vi "myBOT_Draw.vi"(11 "myBOT-Position and Angle":dbl[](array[numeric])) -> (3 "myBOT-Scene":refnum<vi>)   [LabVIEW 2013]
doc: "\"myBOT_Draw.vi\": Draws the myBOT on a 3D Picture Control.\nThis VI has two functions:\n1) The first time the VI is called, CAD Data are gathered, different objects are identified and placed on the 3D Picture Control.\n2) From the second time on the VI is called, the Position (r) and Angle (alpha) are updated.\nThis VI was created for the myRIO Balancing Robot Project. See https://decibel.ni.com/content/groups/myrio-balancing-robot for more information and example projects."
uses:
  <vilib>/picture/3D Picture Control/NI_3D Picture Control.lvlib
panel:
  out "3D Picture Control":refnum<vi>(3d-picture)
  out "Unstable?":bool
  in  "Reset?":bool
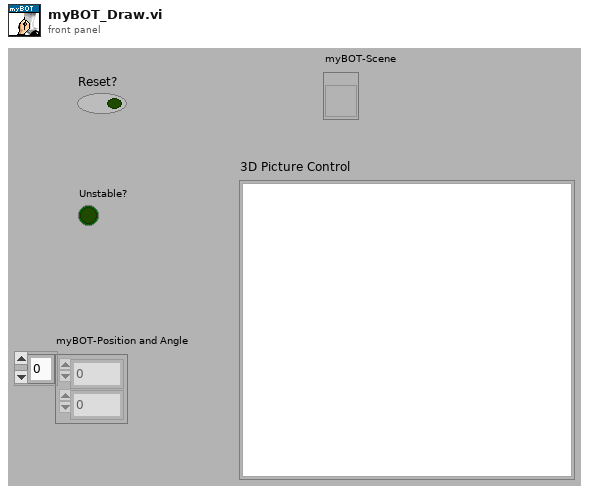
[diagram p1: front panel]
types:
  T1 = enum16{"Inherit Material", "Use entire Material", "Ignore Ambient", "Ignore Diffuse", "Ignore Specular", "Ignore Emission", "Ignore Ambient and Diffuse"}
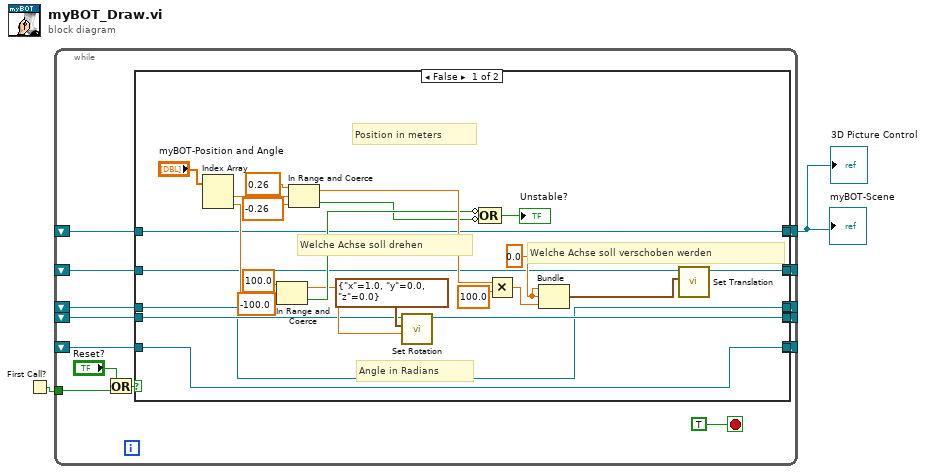
[diagram p0: block diagram]
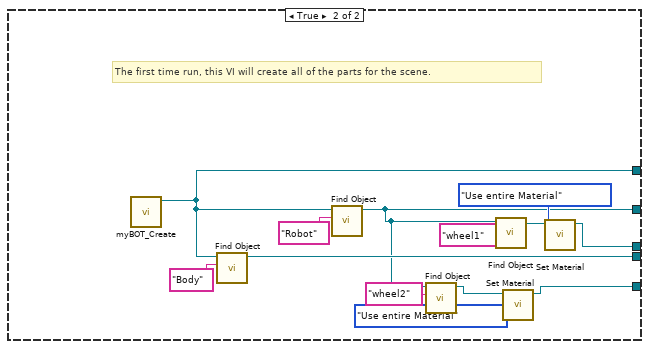
[diagram p2: hidden frame]
diagram:
  n1 = First Call?() -> (First Call?: T/F=w2:bool)
  n2 = while {
    shift-right: [w8] -> w1
    shift-left: _ -> [w7]
    shift-right: [w15] -> _
    shift-left: _ -> [w14]
    shift-right: [w13] -> _
    shift-left: _ -> [w12]
    tunnel: w2 -> [w9]
    shift-right: [w5] -> _
    shift-left: _ -> [w3]
    shift-right: [w6] -> _
    shift-left: _ -> [w4]
    stop <- TRUE stop-if-true
    n3 = Or(x="Reset?", y=w9) -> (x .or. y?=w11:bool)
    n4 = case shown="False" w11 {
      tunnel: [w24 w41] -> w15
      tunnel: w14 -> [w17 _]
      tunnel: [w25 w51] -> w13
      tunnel: w12 -> [w26 _]
      tunnel: [w23 w50] -> w8
      tunnel: w7 -> [w23 _]
      tunnel: [w21 w47] -> w6
      tunnel: [w20 w44] -> w5
      tunnel: w4 -> [w21 _]
      tunnel: w3 -> [w20 _]
      frame False {
        w19 = 0.0
        # "Welche Achse soll verschoben werden"
        # "Welche Achse soll drehen"
        # "Position in meters"
        # "Angle in Radians"
        n5 = Index Array(array="myBOT-Position and Angle") -> (element #1=w34:dbl, element #2=w39:dbl)  [unwired: 2 in]
        n6 = In Range and Coerce(upper limit=100.0, x=w39, lower limit=-100.0) -> (coerced(x)=w28:dbl, In Range?=w31:bool)
        n7 = In Range and Coerce(upper limit=0.26, x=w34, lower limit=-0.26) -> (coerced(x)=w32:dbl, In Range?=w30:bool)
        n8 = call <vilib>:"Set Rotation.vi"("Angle"=w28, "Axis"=cluster{"x":dbl, "y":dbl, "z":dbl} {"x"=1.0, "y"=0.0, "z"=0.0}, "Scene Object"=w26) -> ("Rotated Scene Object"=w25:refnum<vi>)  [unwired: 1 in, 7 out]
        n9 = Compound Arithmetic op=OR(invert w31, invert w30) -> (→"Unstable?":bool)
        n10 = Multiply(x=w32, y=100.0) -> (x*y=w18:dbl)
        n11 = Bundle(w19, w19, w18) -> (w22:cluster{dbl, dbl, dbl})  [unwired: 1 out]
        n12 = call <vilib>:"Set Translation.vi"("Translation"=w22, "Scene Object"=w17) -> ("Translated Object"=w24:refnum<vi>)  [unwired: 1 in, 8 out]
      }
      frame True {
        # "The first time run, this VI will create all of the parts for the scene."
        n13 = call "myBOT_Create.vi"() -> ("SceneObject out"=w50:refnum<vi>)  [unwired: 10 in, 1 out]
        n14 = call <vilib>:"Find Object.vi"("Object Name"="Body" ("Name"), "Scene Refnum"=w50) -> ("Object Refnum"=w51:refnum<vi>)  [unwired: 1 in, 8 out]
        n15 = call <vilib>:"Find Object.vi"("Object Name"="Robot" ("Name"), "Scene Refnum"=w50) -> ("Object Refnum"=w41:refnum<vi>)  [unwired: 1 in, 8 out]
        n16 = call <vilib>:"Find Object.vi"("Object Name"="wheel2", "Scene Refnum"=w41) -> ("Object Refnum"=w43:refnum<vi>)  [unwired: 1 in, 8 out]
        n17 = call <vilib>:"Find Object.vi"("Object Name"="wheel1", "Scene Refnum"=w41) -> ("Object Refnum"=w46:refnum<vi>)  [unwired: 1 in, 8 out]
        n18 = call <vilib>:"Set Material.vi"("Color Mode"=T1."Use entire Material", "Scene Object In"=w43) -> ("Scene Object Out"=w44:refnum<vi>)  [unwired: 8 in, 1 out]
        n19 = call <vilib>:"Set Material.vi"("Color Mode"=T1."Use entire Material", "Scene Object In"=w46) -> ("Scene Object Out"=w47:refnum<vi>)  [unwired: 8 in, 1 out]
      }
    }
  }
  "myBOT-Scene" <- w1
  "3D Picture Control" <- w1
